vi "Create Message.vi"(1 "Message Body":string, 2 "Message Header":string) -> (0 "Message to Send":string)   [LabVIEW 2013]
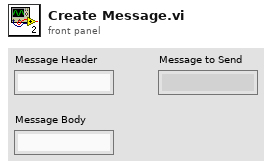
[diagram p1: front panel]
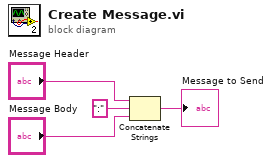
[diagram p0: block diagram]
diagram:
  n1 = Concatenate Strings("Message Header", ":", "Message Body") -> (→"Message to Send":string)
